vi "Connect.vi"(8 "error in (no error)":errorcluster, 11 "DataReceiver in":refnum<class "DataReceiver.lvclass">) -> (0 "error out":errorcluster, 3 "DataReceiver out":refnum<class "DataReceiver.lvclass">)   [LabVIEW 2010, in "DataReceiver.lvclass"]
uses:
  DataReceiver.lvclass
  DataReceiver.lvclass/DataReceiver.ctl
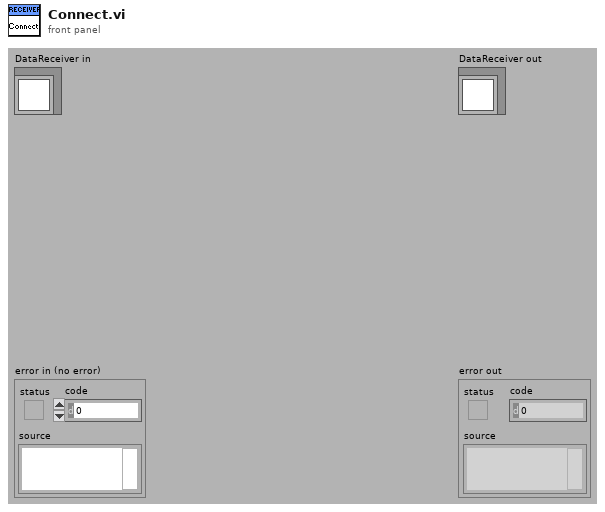
[diagram p1: front panel]
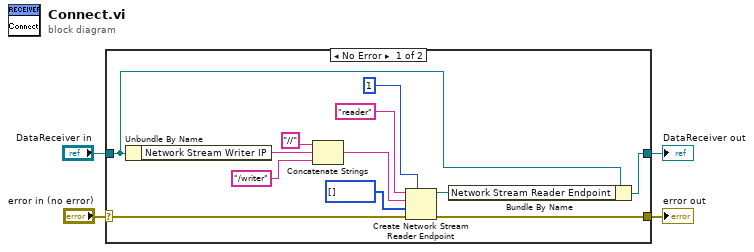
[diagram p0: block diagram]
diagram:
  n1 = case shown="No Error" "error in (no error)" {
    selector: "error in (no error)" -> [w9 w18]
    tunnel: [w8 w18] -> w3
    tunnel: [w6 w17] -> w1
    tunnel: "DataReceiver in" -> [w7 w17]
    frame No Error {
      n2 = Unbundle By Name(w7) -> ("Network Stream Writer IP"=w10:string)
      n3 = Concatenate Strings("//" ("reader url"), w10, "/writer" ("string")) -> (w11:string)
      n4 = Create Network Stream Reader Endpoint(7:1 ("reader buffer size"), 8:w9, 9:i32[] [], 10:w11, 11:"reader" ("writer name")) -> (0:w8:errorcluster, 3:w5:refnum<k21>)  [unwired: 1 in]
      n5 = Bundle By Name(cluster=w7, "Network Stream Reader Endpoint"=w5) -> (w6:refnum<class "DataReceiver.lvclass">)
    }
    frame Error {
    }
  }
  "error out" <- w3
  "DataReceiver out" <- w1
